vi "Close.vi"(8 "error in":errorcluster, 11 "gRPC session in":T1) -> (0 "error out":errorcluster, 3 "gRPC session out":T1)   [LabVIEW 2021, in "dcvmDPI_AD7606B_clientImpl.lvlib"]
uses:
  dcvmDPI_AD7606B_clientImpl.lvlib
  <vilib>/gRPC/LabVIEW gRPC Library/Shared/grpcId.ctl
  dcvmDPI_AD7606B_client/dcvmDPI_AD7606B_client.lvlib
  <vilib>/gRPC/LabVIEW gRPC Library/grpc-lvsupport-release.lvlib
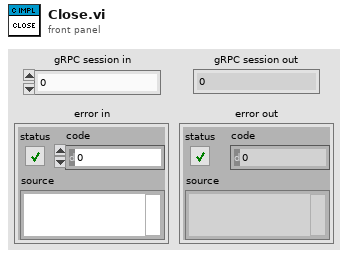
[diagram p1: front panel]
types:
  T1 = typedef "grpc-lvsupport-release.lvlib/grpcId.ctl" = u64
  T2 = typedef "dcvmDPI_AD7606B_client.lvlib/dcvmDPI_CloseResponse.ctl" = cluster{"error":T3}
  T3 = typedef "dcvmDPI_AD7606B_client.lvlib/dcvmDPI_ErrorResponse.ctl" = cluster{"error_number":i32, "error_description":string}
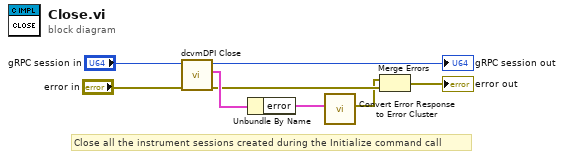
[diagram p0: block diagram]
diagram:
  # "Close all the instrument sessions created during the Initialize command call"
  n1 = call "dcvmDPI Close.vi"("error in"="error in", "gRPC ID"="gRPC session in") -> ("error out"=w3:errorcluster, "Response Data"=w5:T2, "gRPC ID out"=→"gRPC session out":T1)  [unwired: 7 in]
  n2 = Unbundle By Name(w5) -> ("error"=w4:T3)
  n3 = call "Convert Error Response to Error Cluster.vi"("Error response"=w4) -> ("error out"=w2:errorcluster)  [unwired: 10 in]
  n4 = Merge Errors(w2, w3) -> (→"error out":errorcluster)
